vi "pcall_.vi"(4 "nresults":i32, 6 "nargs":i32, 8 "error in (no error)":errorcluster, 11 "Lua in":refnum<class "Lua.lvclass">) -> (0 "error out":errorcluster, 3 "Lua out":refnum<class "Lua.lvclass">)   [LabVIEW 2020, in "Lua for LabVIEW.lvlib" / "Lua.lvclass"]
doc: "Calls a function in protected mode.\n\nTo call a function you must use the following protocol: first, the function to be called is pushed onto the stack; then, the arguments to the function are pushed in direct order; that is, the first argument is pushed first. Finally you call lua_pcall; nargs is the number of arguments that you pushed onto the stack. All arguments and the function value are popped from the stack when the function is called. The function results are pushed onto the stack when the function returns. The number of results is adjusted to nresults, unless nresults is LUA_MULTRET. In this case, all results from the function are pushed. Lua takes care that the returned values fit into the stack space. The function results are pushed onto the stack in direct order (the first result is pushed first), so that after the call the last result is on the top of the stack."
uses:
  Lua.lvclass
  Lua.lvclass/Lua.ctl
  lib/lua.dll/types/lua_error_code_offset.vi
  <vilib>/Utility/error.llb/Error Cluster From Error Code.vi
  lib/lua.dll/lua.dll.lvlib
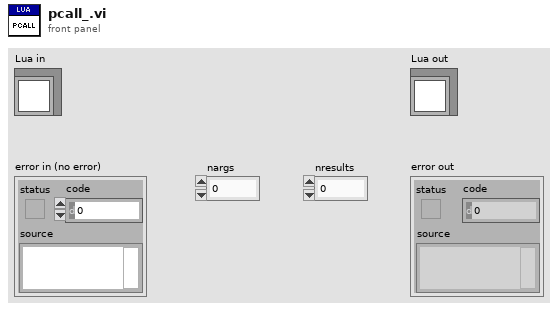
[diagram p1: front panel]
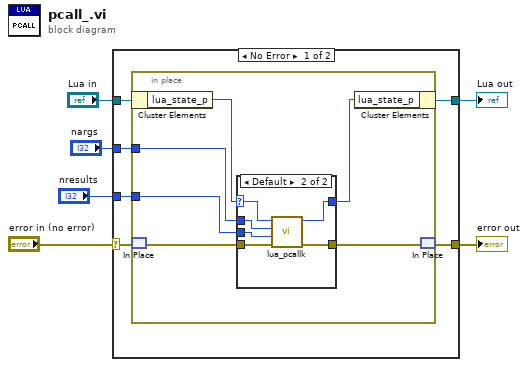
[diagram p0: block diagram]
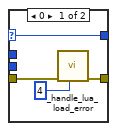
[diagram p2: hidden frame]
diagram:
  n1 = case shown="No Error" "error in (no error)" {
    selector: "error in (no error)" -> [w9 w30]
    tunnel: [w10 w30] -> w3
    tunnel: [w11 w29] -> w6
    tunnel: "Lua in" -> [w12 w29]
    tunnel: "nargs" -> [w8 _]
    tunnel: "nresults" -> [w7 _]
    frame No Error {
      n2 = in-place {
        in-place-border: w8 -> [w14]
        in-place-border: w7 -> [w13]
        n3 = in-place-cluster #1(w12) -> ("lua_state_p"=w17:u64)
        n4 = in-place-match #2(w9) -> (w16:errorcluster)
        n5 = case shown="Default" w17 {
          selector: w17 -> [w22 w24]
          tunnel: [w22 w28] -> w18
          tunnel: w16 -> [w19 w23]
          tunnel: [w20 w25] -> w15
          tunnel: w14 -> [_ w27]
          tunnel: w13 -> [_ w26]
          frame 0 {
            n6 = call "_handle_lua_load_error.vi"("lua_load errcode"=4, "error in (no error)"=w19) -> ("error out"=w20:errorcluster)  [unwired: 9 in]
          }
          frame Default {
            n7 = call "lua_pcallk.vi"("error in (no error)"=w23, "nresults"=w26, "nargs"=w27, "lua_state_p"=w24) -> ("error out"=w25:errorcluster, "lua_state_p out"=w28:u64)  [unwired: 6 in]
          }
        }
        n8 = in-place-cluster #1("lua_state_p"=w18) -> (w11:refnum<class "Lua.lvclass">)
        n9 = in-place-match #2(w15) -> (w10:errorcluster)
      }
    }
    frame Error {
    }
  }
  "error out" <- w3
  "Lua out" <- w6
